vi "TM update all LSC218.vi"(8 "error in (no error)":errorcluster, 11 "VISA Refnum in":refnum<visa-resource-name>) -> (0 "error out":errorcluster, 2 "LSC218 sensors":T1 {"Time stamp" format="%<%H:%M:%S\n%Y/%m/%d>T"}, 3 "VISA Refnum out":refnum<visa-resource-name>)   [LabVIEW 2021, in "Temperature monitor.lvlib"]
doc: "Queries Temperature monitor (LSC218) for all values from sensors in cryostat."
uses:
  Temperature monitor.lvlib
  Typedefs/TM_sensors.ctl
  <instrlib>/Lake Shore Cryotronics 218/Lake Shore Cryotronics 218.lvlib
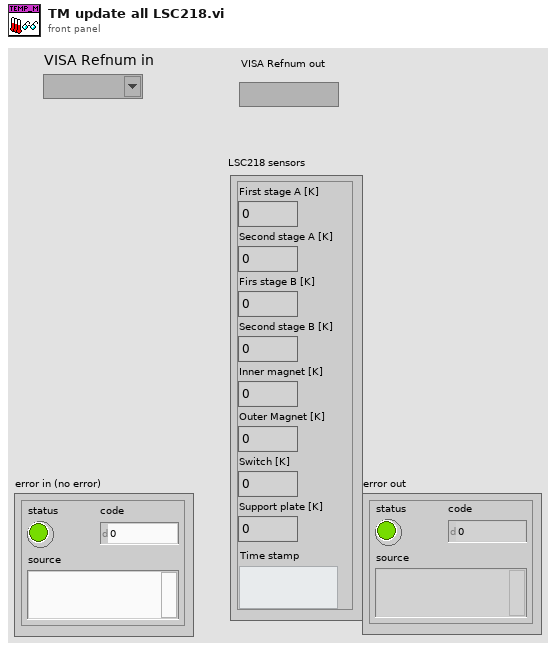
[diagram p1: front panel]
types:
  T1 = typedef "Temperature monitor.lvlib/TM_sensors.ctl" = cluster{"Support plate [K]":dbl, "Switch [K]":dbl, "Outer Magnet [K]":dbl, "Inner magnet [K]":dbl, "Second stage B [K]":dbl, "Firs stage B [K]":dbl, "Second stage A [K]":dbl, "First stage A [K]":dbl, "Time stamp":timestamp}
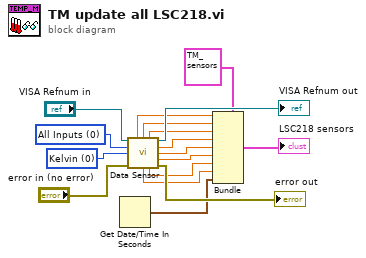
[diagram p0: block diagram]
diagram:
  w2 = u16 0 items=["Kelvin", "Celsius", "Sensor Units", "Linear Data"] ("Data Source (0:Kelvin)")
  w3 = u16 0 items=["All Inputs", "1", "2", "3", "4", "5", "6", "7", "8"] ("Input (0:All)")
  n1 = Get Date/Time In Seconds() -> (seconds since 1Jan1904=w1:timestamp)
  n2 = call <instrlib>:"Data Sensor.vi"("VISA resource name"="VISA Refnum in", "Input (0:All)"=w3, "Data Source (0:Kelvin)"=w2, "error in (no error)"="error in (no error)") -> ("Input 1"=w6:dbl, "Input 2"=w7:dbl, "Input 3"=w8:dbl, "VISA resource name out"=→"VISA Refnum out":refnum<visa-resource-name>, "Input 4"=w9:dbl, "Input 5"=w10:dbl, "Input 6"=w11:dbl, "Input 8"=w13:dbl, "Input 7"=w12:dbl, "error out"=→"error out":errorcluster)  [unwired: 2 in]
  n3 = Bundle(cluster=T1 {"Support plate [K]"=0.0, "Switch [K]"=0.0, "Outer Magnet [K]"=0.0, "Inner magnet [K]"=0.0, "Second stage B [K]"=0.0, "Firs stage B [K]"=0.0, "Second stage A [K]"=0.0, "First stage A [K]"=0.0, "Time stamp"=timestamp(0 s since 1904-01-01)} ("LSC218 sensors"), "Support plate [K]"=w6, "Switch [K]"=w7, "Outer Magnet [K]"=w8, "Inner magnet [K]"=w9, "Second stage B [K]"=w10, "Firs stage B [K]"=w11, "Second stage A [K]"=w12, "First stage A [K]"=w13, "Time stamp"=w1) -> (→"LSC218 sensors":T1)
